vi "loadConfiguration.vi"(8 "error in (no error)":errorcluster, 10 "Load Configuration String in":string, 11 "IDevice in":refnum<class "IDevice.lvclass">) -> (0 "error out":errorcluster, 2 "Load Configuration String out":string, 3 "IDevice out":refnum<class "IDevice.lvclass">)   [LabVIEW 2022 SP3, in "openDAQ.lvlib" / "IBaseObject.lvlib" / "IPropertyObject.lvlib" / "IComponent.lvlib" / "IFolder.lvlib" / "IDevice.lvlib" / "IDevice.lvclass"]
uses:
  <instrlib>/openDAQ/Public/Classes/IDevice/IDevice.lvclass
  <instrlib>/openDAQ/Public/Classes/IDevice/IDevice.lvclass/IDevice.ctl
  <instrlib>/openDAQ/Public/Classes/daqCoreTypes/IString/IString.lvclass
  <instrlib>/openDAQ/Binaries/Windows/x86/copendaq32.dll
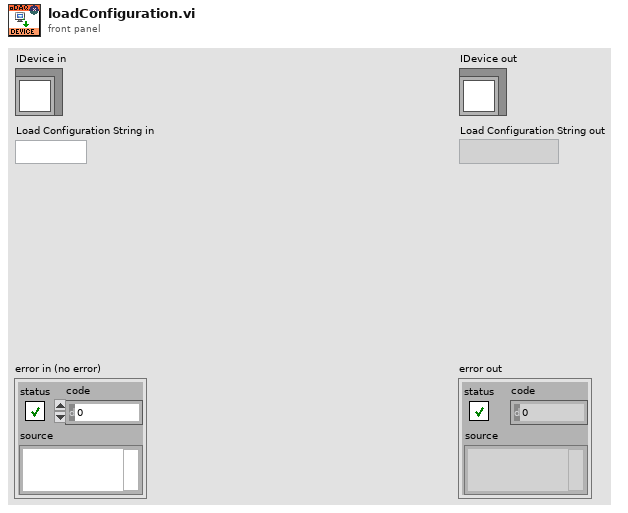
[diagram p1: front panel]
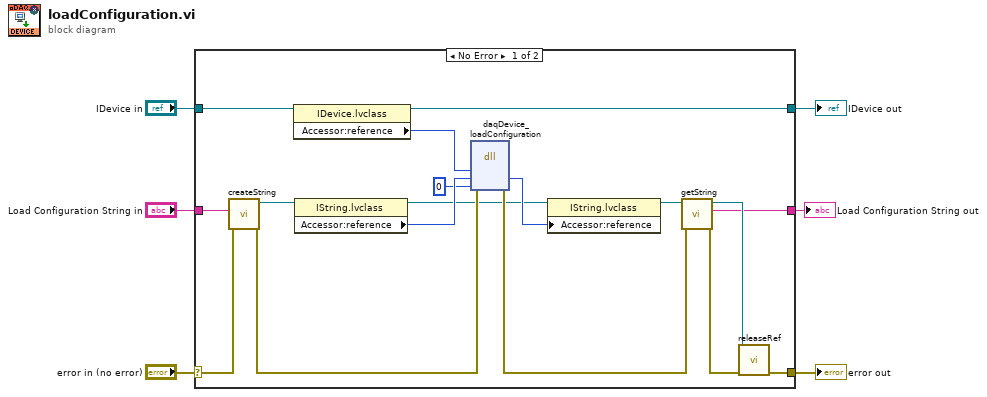
[diagram p0: block diagram]
diagram:
  n1 = case shown="No Error" "error in (no error)" {
    selector: "error in (no error)" -> [w16 w26]
    tunnel: [w13 w26] -> w5
    tunnel: [w20 w25] -> w3
    tunnel: "IDevice in" -> [w22 w25]
    tunnel: "Load Configuration String in" -> [w18 w24]
    tunnel: [w9 w24] -> w1
    frame No Error {
      n2 = call <instrlib>:"createString.vi"("error in (no error)"=w16, "String"=w18) -> ("error out"=w15:errorcluster, "IString out"=w17:refnum<class "IString.lvclass">)  [unwired: 8 in]
      n3 = property class="IDevice.lvclass"(reference=w22) -> (reference out=w20:refnum<class "IDevice.lvclass">, "Accessor:reference"=w21:i64)  [unwired: 1 in, 1 out]
      n4 = property class="IString.lvclass"(reference=w17) -> (reference out=w8:refnum<class "IString.lvclass">, "Accessor:reference"=w19:i64)  [unwired: 1 in, 1 out]
      n5 = dll-call lib="C:/Program Files (x86)/National Instruments/LabVIEW 2022/instr.lib/openDAQ/Binaries/Windows/x86/copendaq*.*" fn="daqDevice_loadConfiguration"(error in=w15, "device"=w21, "configuration"=w19, "updateParameters"=0) -> (error out=w11:errorcluster, "configuration"=w23:i64)  [unwired: 5 in, 1 out]
      n6 = property class="IString.lvclass"(reference=w8, "Accessor:reference"=w23) -> (reference out=w14:refnum<class "IString.lvclass">)  [unwired: 1 in, 1 out]
      n7 = call <instrlib>:"getString.vi"("error in (no error)"=w11, "IString in"=w14) -> ("error out"=w10:errorcluster, "String out"=w9:string, "IString out"=w12:refnum<class "IString.lvclass">)  [unwired: 7 in]
      n8 = call-dynamic "releaseRef.vi"("error in (no error)"=w10, "IBaseObject in"=w12) -> ("error out"=w13:errorcluster)  [unwired: 9 in]
    }
    frame Error {
    }
  }
  "error out" <- w5
  "IDevice out" <- w3
  "Load Configuration String out" <- w1
